vi "Agilent PWM Wait for Operation Complete (OPC) 2.vi"(8 "error in (no error)":errorcluster, 9 "Timeout (300s)":u32=300 max=1000, 10 "Command (*OPC?)":string="*OPC?", 11 "VISA Resource Name":refnum<visa-resource-name>) -> (0 "error out":errorcluster, 2 "Read Buffer":string, 3 "VISA Resource Name Out":refnum<visa-resource-name>)   [LabVIEW 2011]
doc: "This VI send a command to the instrument and waits for the response."
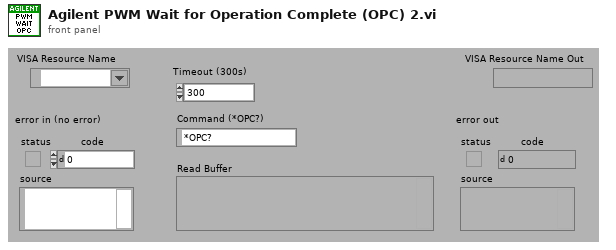
[diagram p1: front panel]
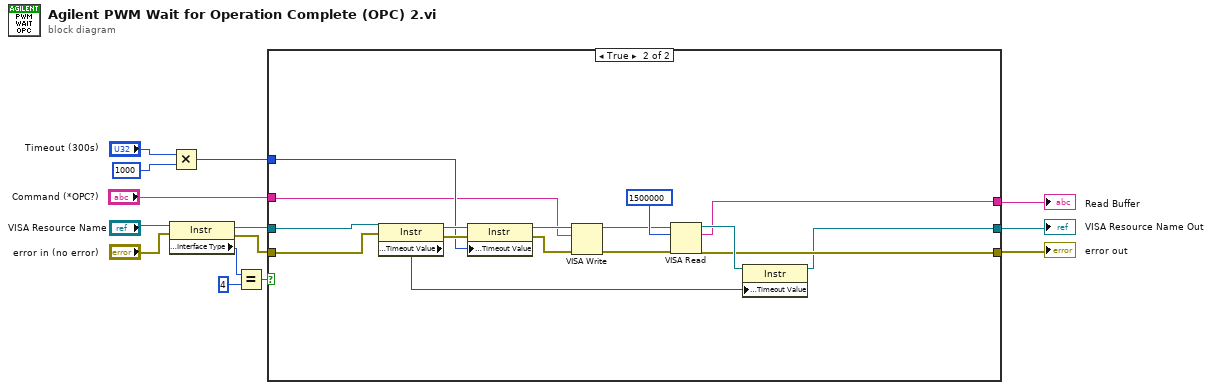
[diagram p0: block diagram]
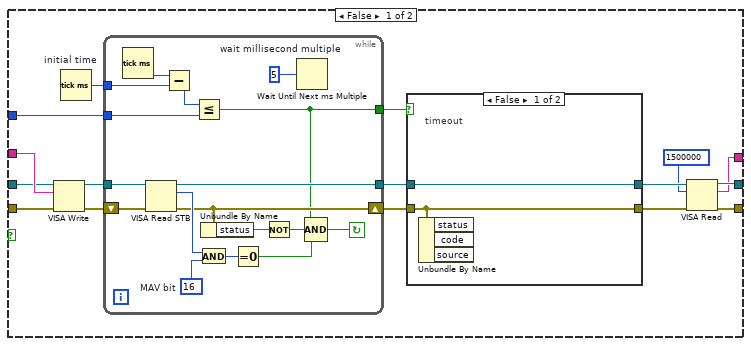
[diagram p2: hidden frame]
diagram:
  n1 = property on="Property Node" class="Instr"(reference="VISA Resource Name", error in="error in (no error)") -> (reference out=w5:refnum<visa-resource-name>, error out=w4:errorcluster, "Interface Information:Interface Type"=w9:u16)
  n2 = Multiply(x="Timeout (300s)", y=u32 1000) -> (x*y=w11:u32)
  n3 = Equal?(x=w9, y=u16 4) -> (x = y?=w3:bool)
  n4 = case shown="True" w3 {
    tunnel: [w20 w57] -> w2
    tunnel: w11 -> [w26 w56]
    tunnel: "Command (*OPC?)" -> [w25 w55]
    tunnel: w4 -> [w24 w58]
    tunnel: w5 -> [w23 w52]
    tunnel: [w17 w53] -> w1
    tunnel: [w16 w54] -> w10
    frame False {
      n5 = VISA Write(VISA resource name=w23, write buffer=w25, error in (no error)=w24) -> (VISA resource name out=w21:refnum<visa-resource-name>, error out=w22:errorcluster)  [unwired: 1 out]
      n6 = Tick Count (ms) "initial time"() -> (millisecond timer value=w27:u32)
      n7 = while {
        tunnel: w21 -> [w46]
        tunnel: [w45] -> w29
        shift-right: [w36] -> w30
        shift-left: w22 -> [w47]
        tunnel: w26 -> [w37]
        tunnel: w27 -> [w39]
        tunnel: [w31] -> w28
        stop <- w33 continue-if-true
        w41 = u32 5  # wait millisecond multiple
        w43 = u16 16  # MAV bit
        n8 = Tick Count (ms)() -> (millisecond timer value=w40:u32)
        n9 = VISA Read STB(8:w47, 11:w46) -> (0:w36:errorcluster, 2:w44:u16, 3:w45:refnum<visa-resource-name>)
        n10 = Subtract(x=w40, y=w39) -> (x-y=w38:u32)
        n11 = Less Or Equal?(x=w38, y=w37) -> (x <= y?=w31:bool)
        n12 = And(x=w44, y=w43) -> (x .and. y?=w42:u16)
        n13 = Unbundle By Name(w36) -> ("status"=w35:bool)
        n14 = Equal To 0?(x=w42) -> (x = 0?=w32:bool)
        n15 = Not(x=w35) -> (.not. x?=w34:bool)
        n16 = Wait Until Next ms Multiple(millisecond multiple=w41) -> ()  [unwired: 1 out]
        n17 = Compound Arithmetic op=AND(w31, w34, w32) -> (w33:bool)
      }
      n18 = case shown="False" w28 {
        tunnel: w29 -> [w48 w51]
        tunnel: w30 -> [w49 w50]
        tunnel: [w49 w50] -> w19
        tunnel: [w48 w51] -> w18
        frame False {
          # "timeout"
          n19 = Unbundle By Name(w49) -> ()  [unwired: 3 out]
        }
        frame True {
          # "no timeout"
        }
      }
      n20 = VISA Read(VISA resource name=w18, byte count=u32 1500000 ("byte count (0)"), error in (no error)=w19) -> (VISA resource name out=w17:refnum<visa-resource-name>, read buffer=w16:string, error out=w20:errorcluster)  [unwired: 1 out]
    }
    frame True {
      n21 = property on="Property Node" class="Instr"(reference=w52, error in=w58) -> (reference out=w67:refnum<visa-resource-name>, error out=w66:errorcluster, "General Settings:Timeout Value"=w63:u32)
      n22 = property on="Property Node" class="Instr"(reference=w67, error in=w66, "General Settings:Timeout Value"=w56) -> (reference out=w65:refnum<visa-resource-name>, error out=w64:errorcluster)
      n23 = VISA Write(VISA resource name=w65, write buffer=w55, error in (no error)=w64) -> (VISA resource name out=w61:refnum<visa-resource-name>, error out=w60:errorcluster)  [unwired: 1 out]
      n24 = VISA Read(VISA resource name=w61, byte count=u32 1500000 ("byte count (0)"), error in (no error)=w60) -> (VISA resource name out=w59:refnum<visa-resource-name>, read buffer=w54:string, error out=w57:errorcluster)  [unwired: 1 out]
      n25 = property on="Property Node" class="Instr"(reference=w59, "General Settings:Timeout Value"=w63) -> (reference out=w53:refnum<visa-resource-name>)  [unwired: 1 in, 1 out]
    }
  }
  "error out" <- w2
  "VISA Resource Name Out" <- w1
  "Read Buffer" <- w10
